vi "麻醉眼位置记录.vi"() -> ()   [LabVIEW 2011]
uses:
  <vilib>/Analysis/NI_AALBase.lvlib
panel:
  out "eye1 2":T1(graph)
  in  "recording bin":i32=400
  in  "bin":i32=250
  out "eye1":T1(graph)
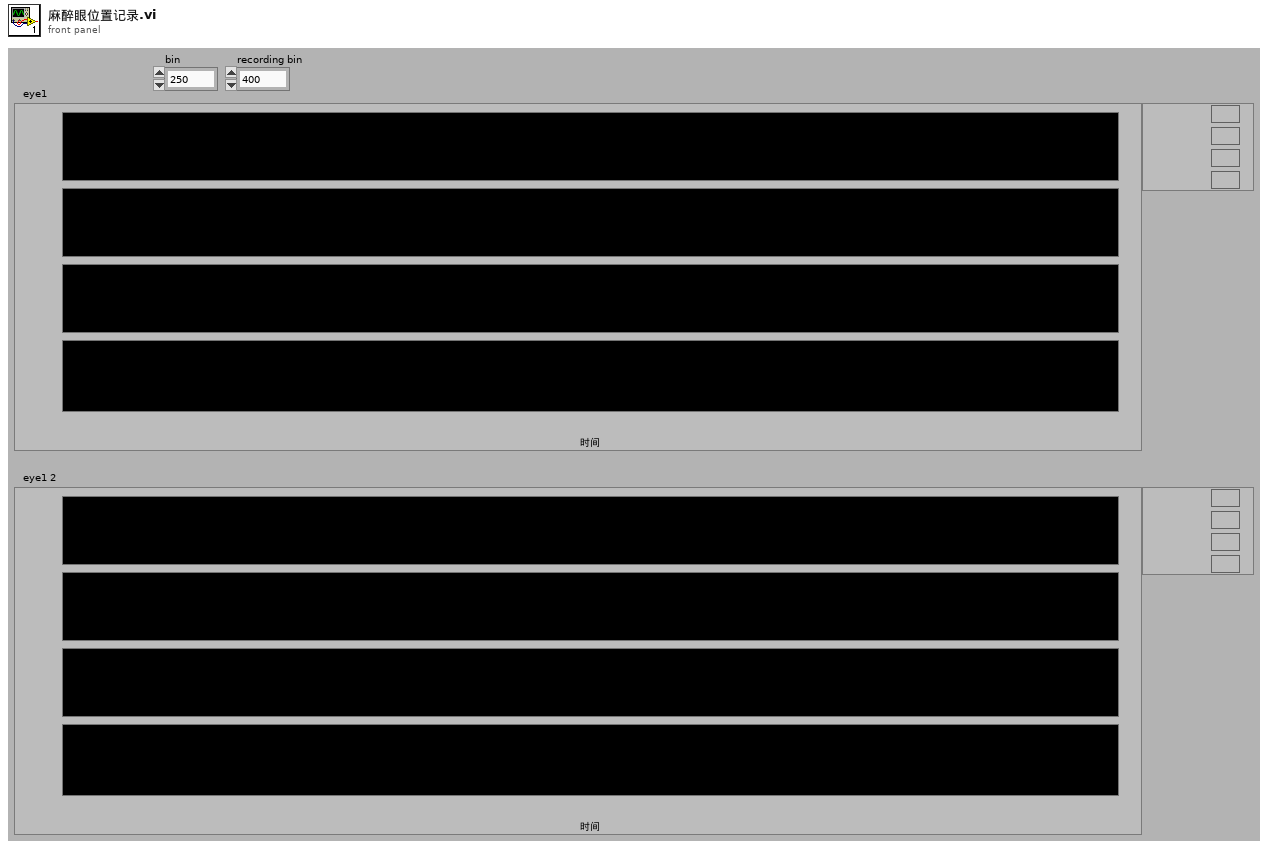
[diagram p1: front panel]
types:
  T1 = cluster{"mean":dbl, "mean":dbl, "mean":dbl, "mean":dbl}
  T2 = enum16{"open", "replace", "create", "open or create", "replace or create", "replace or create with confirmation"}
  T3 = cluster{"mean":dbl, "mean":dbl, "mean":dbl, "mean":dbl}[]
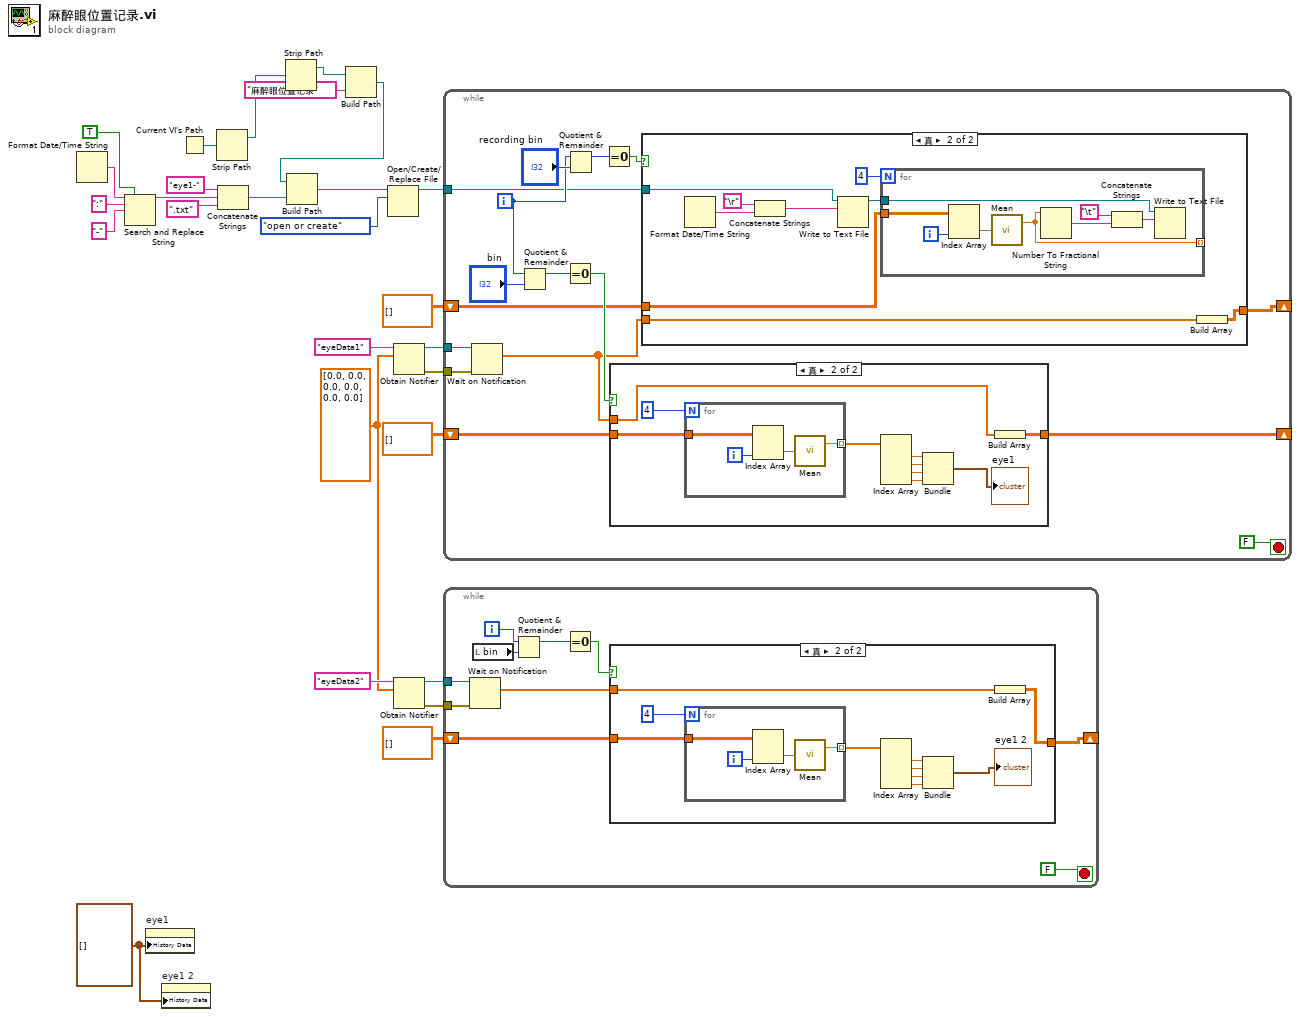
[diagram p0: block diagram]
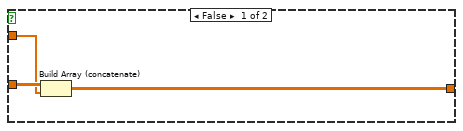
[diagram p2: hidden frame]
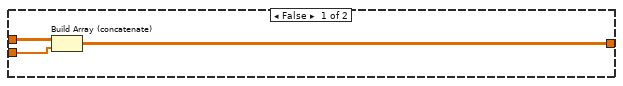
[diagram p3: hidden frame]
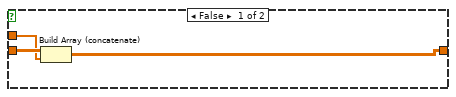
[diagram p4: hidden frame]
diagram:
  w5 = T3 [] ("历史数据")
  w23 = dbl[] [0.0, 0.0, 0.0, 0.0, 0.0, 0.0] ("添加的数组")
  n1 = Format Date/Time String() -> (date/time string=w9:string)  [unwired: 3 out]
  n2 = Search and Replace String(replace all?=TRUE ("替换全部？(F)"), input string=w9, search string=":" ("搜索字符串"), replace string="-" ("替换字符串(\"\")")) -> (result string=w6:string)  [unwired: 1 in, 6 out]
  n3 = property on="eye1" class="WFChart (严格)"("History Data"=w5) -> ()  [unwired: 2 in, 2 out]
  n4 = property on="eye1 2" class="WFChart (严格)"("History Data"=w5) -> ()  [unwired: 2 in, 2 out]
  n5 = Current VI's Path() -> (path=w17:path)
  n6 = Strip Path(path=w17) -> (stripped path=w4:path)  [unwired: 1 out]
  n7 = Concatenate Strings("eye1-" ("名称或相对路径"), w6, ".txt" ("名称或相对路径")) -> (w11:string)
  n8 = Strip Path(path=w4) -> (stripped path=w3:path)  [unwired: 1 out]
  n9 = Build Path(base path=w3, name or relative path="麻醉眼位置记录" ("名称或相对路径")) -> (appended path=w1:path)
  n10 = Build Path(base path=w1, name or relative path=w11) -> (appended path=w14:path)
  n11 = Open/Create/Replace File(file path (use dialog)=w14, operation (0:open)=T2."open or create" ("操作(0:open)")) -> (refnum out=w15:refnum<file>)  [unwired: 1 in, 5 out]
  n12 = Obtain Notifier(name (unnamed)="eyeData1" ("Image Name"), notification data type=w23) -> (notifier out=w26:refnum<notifier>, error out=w25:errorcluster)  [unwired: 2 in, 1 out]
  n13 = Obtain Notifier(name (unnamed)="eyeData2" ("Image Name"), notification data type=w23) -> (notifier out=w21:refnum<notifier>, error out=w20:errorcluster)  [unwired: 2 in, 1 out]
  n14 = while {
    tunnel: w26 -> [w43]
    tunnel: w25 -> [w42]
    shift-right: [w37] -> _
    shift-left: dbl[][] [] -> [w36]
    shift-right: [w35] -> _
    shift-left: dbl[][] [] -> [w34]
    tunnel: w15 -> [w28]
    i -> [w30]
    stop <- FALSE stop-if-true
    n15 = Wait on Notification(notifier=w43, error in (no error)=w42) -> (notification=w33:dbl[])  [unwired: 5 out]
    n16 = Quotient & Remainder(x=w30, y="bin") -> (x-y*floor(x/y)=w39:i32)  [unwired: 1 out]
    n17 = Equal To 0?(x=w39) -> (x = 0?=w38:bool)
    n18 = Quotient & Remainder(x=w30, y="recording bin") -> (x-y*floor(x/y)=w32:i32)  [unwired: 1 out]
    n19 = Equal To 0?(x=w32) -> (x = 0?=w29:bool)
    n20 = case shown="真" w38 {
      tunnel: [w65 w75] -> w37
      tunnel: w36 -> [w66 w73]
      tunnel: w33 -> [w64 w76]
      frame False {
        n21 = Build Array (concatenate)(w66, w64) -> (w65:dbl[][])
      }
      frame True {
        n22 = for {
          N: 4 -> [_]
          tunnel: [w80] -> w72 mode=indexing
          tunnel: w73 -> [w79]
          i -> [w78]
          n23 = Index Array(array=w79, index (col)=w78) -> (element=w77:dbl[])  [unwired: 1 in]
          n24 = call <vilib>:"Mean.vi"("X"=w77) -> ("mean"=w80:dbl)  [unwired: 1 out]
        }
        n25 = Index Array(array=w72) -> (element #1=w71:dbl, element #2=w70:dbl, element #3=w69:dbl, element #4=w68:dbl)  [unwired: 4 in]
        n26 = Bundle("mean"=w71, "mean"=w70, "mean"=w69, "mean"=w68) -> (→"eye1":T1)  [unwired: 1 out]
        n27 = Build Array(w76) -> (w75:dbl[][])
      }
    }
    n28 = case shown="真" w29 {
      tunnel: [w45 w54] -> w35
      tunnel: w34 -> [w46 w52]
      tunnel: w33 -> [w44 w55]
      tunnel: w28 -> [_ w51]
      frame False {
        n29 = Build Array (concatenate)(w46, w44) -> (w45:dbl[][])
      }
      frame True {
        n30 = Format Date/Time String() -> (date/time string=w49:string)  [unwired: 3 out]
        n31 = Concatenate Strings("\r", w49) -> (w47:string)
        n32 = Write to Text File(file (use dialog)=w51, text=w47) -> (refnum out=w48:refnum<file>)  [unwired: 1 in, 3 out]
        n33 = for {
          N: 4 -> [_]
          tunnel: [w60] -> _ mode=indexing
          tunnel: w52 -> [w63]
          tunnel: w48 -> [w58]
          i -> [w62]
          n34 = Index Array(array=w63, index (col)=w62) -> (element=w61:dbl[])  [unwired: 1 in]
          n35 = call <vilib>:"Mean.vi"("X"=w61) -> ("mean"=w60:dbl)  [unwired: 1 out]
          n36 = Number To Fractional String(number=w60) -> (F-format string=w56:string)  [unwired: 3 out]
          n37 = Concatenate Strings("\t", w56) -> (w59:string)
          n38 = Write to Text File(file (use dialog)=w58, text=w59) -> ()  [unwired: 1 in, 4 out]
        }
        n39 = Build Array(w55) -> (w54:dbl[][])
      }
    }
  }
  n40 = while {
    tunnel: w21 -> [w90]
    tunnel: w20 -> [w89]
    shift-right: [w84] -> _
    shift-left: dbl[][] [] -> [w83]
    i -> [w87]
    stop <- FALSE stop-if-true
    n41 = Wait on Notification(notifier=w90, error in (no error)=w89) -> (notification=w82:dbl[])  [unwired: 5 out]
    n42 = local read "bin"() -> (w81:i32)
    n43 = Quotient & Remainder(x=w87, y=w81) -> (x-y*floor(x/y)=w86:i32)  [unwired: 1 out]
    n44 = Equal To 0?(x=w86) -> (x = 0?=w85:bool)
    n45 = case shown="真" w85 {
      tunnel: [w92 w102] -> w84
      tunnel: w83 -> [w93 w100]
      tunnel: w82 -> [w91 w103]
      frame False {
        n46 = Build Array (concatenate)(w93, w91) -> (w92:dbl[][])
      }
      frame True {
        n47 = for {
          N: 4 -> [_]
          tunnel: [w107] -> w99 mode=indexing
          tunnel: w100 -> [w106]
          i -> [w105]
          n48 = Index Array(array=w106, index (col)=w105) -> (element=w104:dbl[])  [unwired: 1 in]
          n49 = call <vilib>:"Mean.vi"("X"=w104) -> ("mean"=w107:dbl)  [unwired: 1 out]
        }
        n50 = Index Array(array=w99) -> (element #1=w98:dbl, element #2=w97:dbl, element #3=w96:dbl, element #4=w95:dbl)  [unwired: 4 in]
        n51 = Bundle("mean"=w98, "mean"=w97, "mean"=w96, "mean"=w95) -> (→"eye1 2":T1)  [unwired: 1 out]
        n52 = Build Array(w103) -> (w102:dbl[][])
      }
    }
  }
